vi "Create Message.vi"(7 "App":refnum<vi>, 8 "error in (no error)":errorcluster, 10 "Message":T1, 11 "LV-Protoc in":refnum<class "LV-Protoc.lvclass">) -> (0 "error out":errorcluster, 2 "Missing Deps":bool, 3 "LV-Protoc out":refnum<class "LV-Protoc.lvclass">)   [LabVIEW 2020, in "LV-Protoc.lvlib" / "LV-Protoc.lvclass"]
uses:
  LV-Protoc.lvclass
  LV-Proto/Message.ctl
  LV-Proto/Field.ctl
  LV-Proto/Type.ctl
  LV-Proto/Proto Type.ctl
  LV-Proto/LV-Proto.lvlib
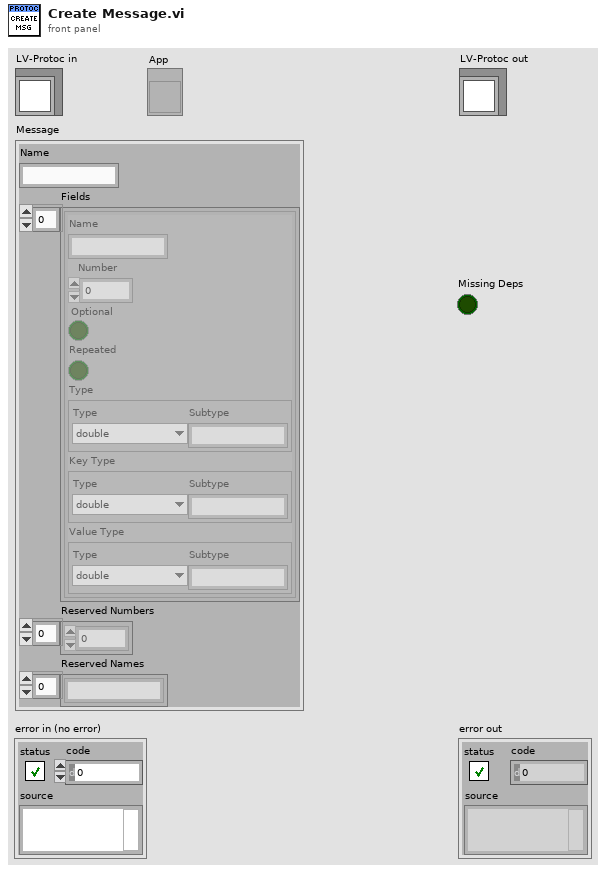
[diagram p1: front panel]
types:
  T1 = typedef "LV-Proto.lvlib/Message.ctl" = cluster{"Name":string, "Fields":T2[], "Reserved Numbers":u32[], "Reserved Names":string[]}
  T2 = typedef "LV-Proto.lvlib/Field.ctl" = cluster{"Name":string, "Number":u32, "Optional":bool, "Repeated":bool, "Type":T3, "Key Type":T3, "Value Type":T3}
  T3 = typedef "LV-Proto.lvlib/Type.ctl" = cluster{"Type":T4, "Subtype":string}
  T4 = typedef "LV-Proto.lvlib/Proto Type.ctl" = enum16{"UNKNOWN", "double", "float", "int32", "int64", "uint32", "uint64", "sint32", "sint64", "fixed32", "fixed64", "sfixed32", "sfixed64", "bool", "string", "bytes", "enum", "map", "message"}
  T5 = typedef "LV-Protoc.lvlib/Message Paths.ctl" = cluster{"Name":string, "Library":path, "Data Typedef":path, "MessageName VI":path, "Flatten VI":path, "Unflatten VI":path, "Flatten repeated VI":path, "Decode VI":path}
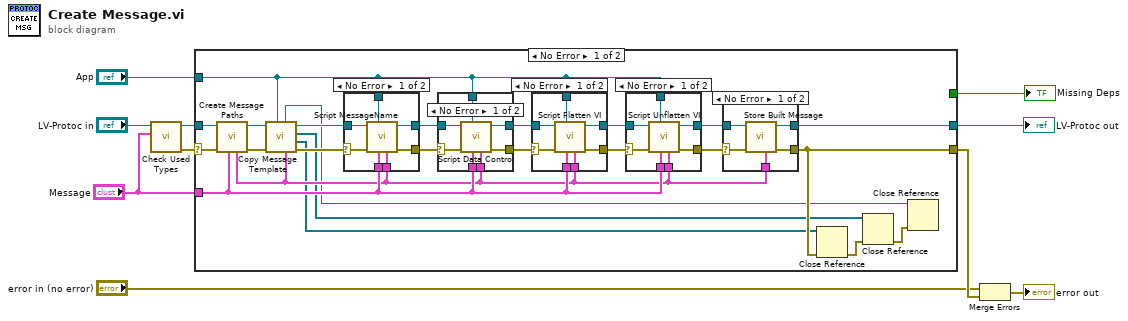
[diagram p0: block diagram]
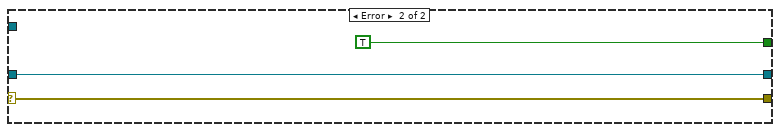
[diagram p7: hidden frame]
diagram:
  n1 = call "Check Used Types.vi"("Message"="Message", "LV-Protoc in"="LV-Protoc in") -> ("error out"=w9:errorcluster, "LV-Protoc out"=w8:refnum<class "LV-Protoc.lvclass">)  [unwired: 8 in]
  n2 = case shown="No Error" w9 {
    selector: w9 -> [w31 w80]
    tunnel: w8 -> [w33 w79]
    tunnel: [w34 w80] -> w6
    tunnel: "Message" -> [w18 _]
    tunnel: [w24 w79] -> w3
    tunnel: [_ TRUE] -> w2
    tunnel: "App" -> [w16 _]
    frame No Error {
      n3 = call "Create Message Paths.vi"("Message"=w18, "error in (no error)"=w31, "LV-Protoc in"=w33) -> ("error out"=w30:errorcluster, "LV-Protoc out"=w32:refnum<class "LV-Protoc.lvclass">, "Message Paths"=w17:T5)  [unwired: 6 in]
      n4 = call "Copy Message Template.vi"("Message Paths"=w17, "App"=w16, "error in (no error)"=w30, "LV-Protoc in"=w32) -> ("error out"=w21:errorcluster, "Nested Libraries"=w15:refnum<vi>[], "VIs"=w13:refnum<vi>[], "LV-Protoc out"=w22:refnum<class "LV-Protoc.lvclass">, "Library"=w12:refnum<vi>)  [unwired: 3 in]
      n5 = case shown="No Error" w21 {
        selector: w21 -> [w39 w42]
        tunnel: w22 -> [w41 w43]
        tunnel: [w40 w43] -> w19
        tunnel: w18 -> [w38 _]
        tunnel: w17 -> [w37 _]
        tunnel: [w36 w42] -> w20
        tunnel: w16 -> [w35 _]
        frame No Error {
          n6 = call "Script MessageName.vi"("Message Paths"=w37, "Message"=w38, "App"=w35, "error in (no error)"=w39, "LV-Protoc in"=w41) -> ("error out"=w36:errorcluster, "LV-Protoc out"=w40:refnum<class "LV-Protoc.lvclass">)  [unwired: 5 in]
        }
        frame Error {
        }
      }
      n7 = case shown="No Error" w20 {
        selector: w20 -> [w73 w76]
        tunnel: w19 -> [w75 w77]
        tunnel: [w74 w77] -> w29
        tunnel: w18 -> [w72 _]
        tunnel: w17 -> [w71 _]
        tunnel: [w70 w76] -> w28
        tunnel: w16 -> [w69 _]
        frame No Error {
          n8 = call "Script Data Control.vi"("Message Paths"=w71, "Message"=w72, "App"=w69, "error in (no error)"=w73, "LV-Protoc in"=w75) -> ("error out"=w70:errorcluster, "LV-Protoc out"=w74:refnum<class "LV-Protoc.lvclass">)  [unwired: 5 in]
        }
        frame Error {
        }
      }
      n9 = case shown="No Error" w28 {
        selector: w28 -> [w64 w67]
        tunnel: w29 -> [w66 w68]
        tunnel: [w65 w68] -> w26
        tunnel: w18 -> [w63 _]
        tunnel: w17 -> [w62 _]
        tunnel: [w61 w67] -> w27
        tunnel: w16 -> [w60 _]
        frame No Error {
          n10 = call "Script Flatten VI.vi"("Message Paths"=w62, "Message"=w63, "App"=w60, "error in (no error)"=w64, "LV-Protoc in"=w66) -> ("error out"=w61:errorcluster, "LV-Protoc out"=w65:refnum<class "LV-Protoc.lvclass">)  [unwired: 5 in]
        }
        frame Error {
        }
      }
      n11 = case shown="No Error" w27 {
        selector: w27 -> [w55 w58]
        tunnel: w26 -> [w57 w59]
        tunnel: [w56 w59] -> w25
        tunnel: w18 -> [w54 _]
        tunnel: w17 -> [w53 _]
        tunnel: [w52 w58] -> w23
        tunnel: w16 -> [w51 _]
        frame No Error {
          n12 = call "Script Unflatten VI.vi"("Message Paths"=w53, "Message"=w54, "App"=w51, "error in (no error)"=w55, "LV-Protoc in"=w57) -> ("error out"=w52:errorcluster, "LV-Protoc out"=w56:refnum<class "LV-Protoc.lvclass">)  [unwired: 5 in]
        }
        frame Error {
        }
      }
      n13 = case shown="No Error" w23 {
        selector: w23 -> [w47 w50]
        tunnel: [w48 w49] -> w24
        tunnel: w17 -> [w46 _]
        tunnel: [w45 w50] -> w34
        tunnel: w25 -> [w44 w49]
        frame No Error {
          n14 = call "Store Built Message.vi"("Message Paths"=w46, "error in (no error)"=w47, "LV-Protoc in"=w44) -> ("error out"=w45:errorcluster, "LV-Protoc out"=w48:refnum<class "LV-Protoc.lvclass">)  [unwired: 7 in]
        }
        frame Error {
        }
      }
      n15 = Close Reference(reference=w15, error in (no error)=w34) -> (error out=w14:errorcluster)
      n16 = Close Reference(reference=w13, error in (no error)=w14) -> (error out=w11:errorcluster)
      n17 = Close Reference(reference=w12, error in (no error)=w11) -> ()  [unwired: 1 out]
    }
    frame Error {
    }
  }
  "LV-Protoc out" <- w3
  "Missing Deps" <- w2
  n18 = Merge Errors("error in (no error)", w6) -> (→"error out":errorcluster)
